vi "AnalogCNTL_MKS.vi"() -> ()   [LabVIEW 2015]
uses:
  <userlib>/caLab/Private/Get_PV-1D.vi
panel:
  in  "LocalEpics":u16(ring) items=["LOCAL", "EPCIS"]
  out "APX:HPC100":dbl format="%.3g"
  out "APX:HPC01":dbl format="%_6g"
  out "Gain":dbl format="%#_6f"
  out "Vin":dbl
  in  "Vref":dbl min=0.0 max=5.0 step=0.01
  in  "ManualAuto":u16(ring) items=["CLOSE", "OPEN", "AUTO"]
  in  "MFC0:Pcell_RQ":dbl
  out "MFC0:Pcell":dbl
  in  "stop":bool
  # "MFC0"
  # "MFC"
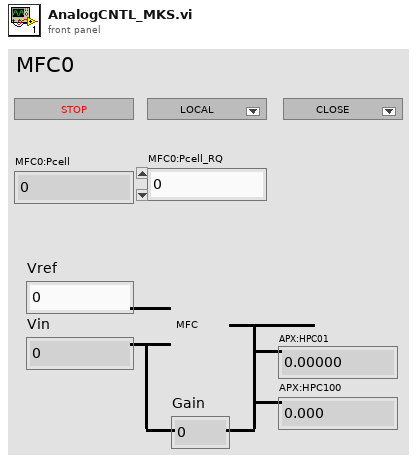
[diagram p1: front panel]
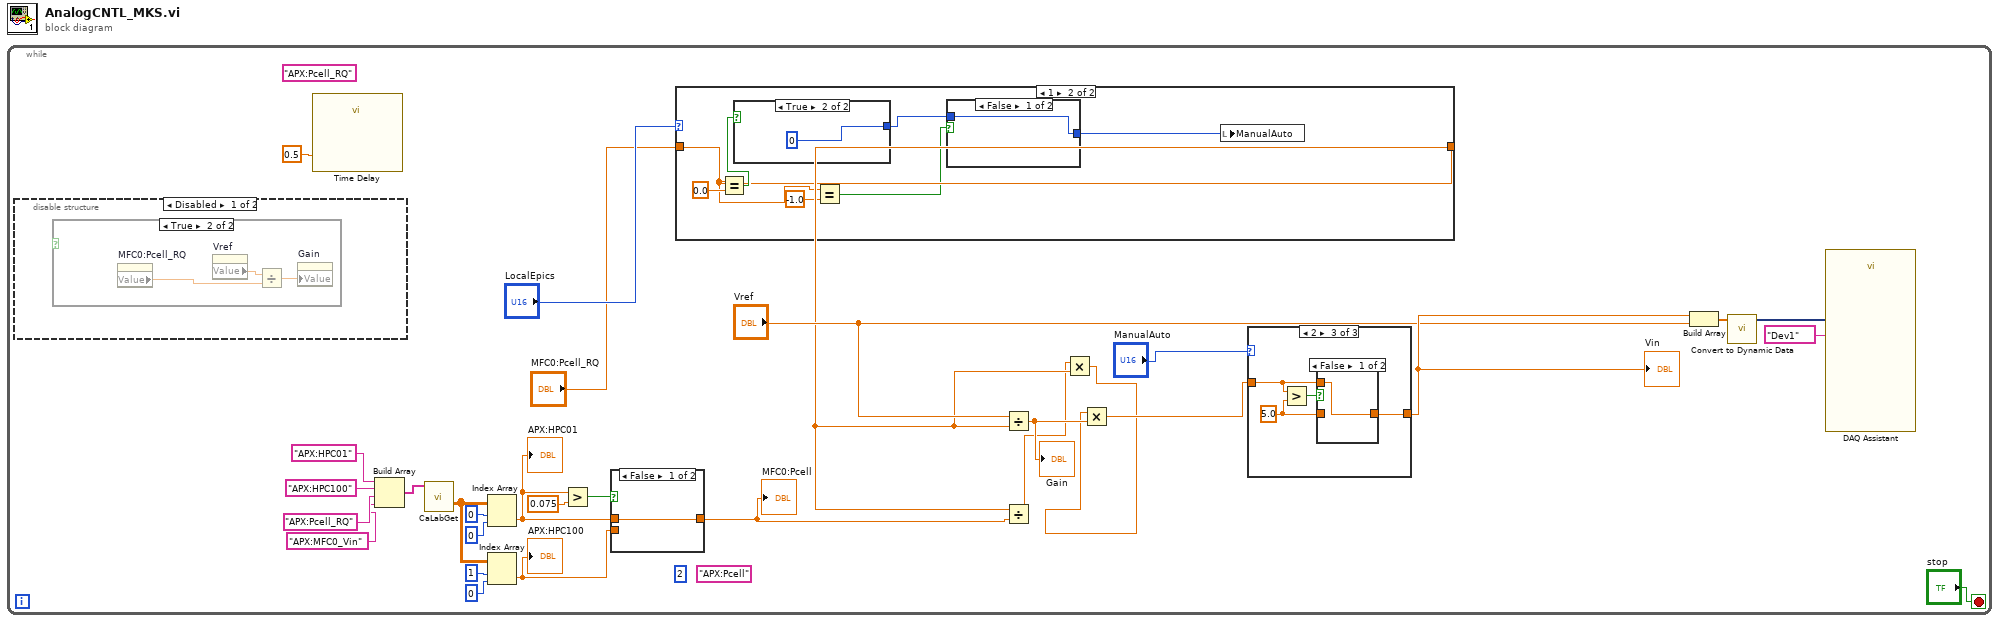
[diagram p0: block diagram]
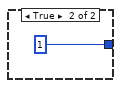
[diagram p4: hidden frame]
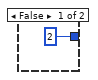
[diagram p5: hidden frame]
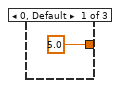
[diagram p8: hidden frame]
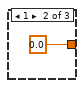
[diagram p9: hidden frame]
diagram:
  n1 = while {
    stop <- "stop" stop-if-true
    (unwired) "APX:Pcell"
    (unwired) "APX:Pcell_RQ"
    (unwired) u16 2 ("y")
    n2 = disable-structure shown="Disabled" {
      frame Disabled {
        n3 = case shown="True" {
          selector: _ -> [_ _]
          frame False {
          }
          frame True {
            n4 = property on="MFC0:Pcell_RQ" class="DigNum (strict)"() -> ("Value"=w45:dbl)  [unwired: 2 in, 2 out]
            n5 = property on="Vref" class="DigNum (strict)"() -> ("Value"=w46:dbl)  [unwired: 2 in, 2 out]
            n6 = Divide(x=w46, y=w45) -> (x/y=w47:dbl)
            n7 = property on="Gain" class="DigNum (strict)"("Value"=w47) -> ()  [unwired: 2 in, 2 out]
          }
        }
      }
      frame Enabled {
      }
    }
    n8 = call "Time Delay"("Delay Time (s)"=0.5) -> ()  [unwired: 10 in, 1 out]
    n9 = Build Array("APX:HPC01", "APX:HPC100", "APX:Pcell_RQ", "APX:MFC0_Vin") -> (w24:string[])
    n10 = call-poly "CaLabGet.vi"("PV Names"=w24) -> ("Value Array (number)"=w20:dbl[][])  [unwired: 8 in, 6 out]
    n11 = Index Array(array=w20, index (row)=0 ("disabled index (col)"), index (col)=0) -> (element=w10:dbl)
    "APX:HPC01" <- w10
    n12 = Index Array(array=w20, index (row)=1 ("disabled index (col)"), index (col)=0) -> (element=w11:dbl)
    "APX:HPC100" <- w11
    n13 = Greater?(x=w10, y=0.075) -> (0:w13:bool)
    n14 = case shown="False" w13 {
      tunnel: w11 -> [_ w32]
      tunnel: [w31 w32] -> w5
      tunnel: w10 -> [w31 _]
      frame False {
      }
      frame True {
      }
    }
    "MFC0:Pcell" <- w5
    n15 = case shown="1" "LocalEpics" {
      tunnel: "MFC0:Pcell_RQ" -> [w33 w37]
      tunnel: [w33 w37] -> w3
      frame 0, Default {
      }
      frame 1 {
        n16 = Equal?(x=w37, y=0.0) -> (x = y?=w38:bool)
        n17 = case shown="True" w38 {
          tunnel: [u16 2 ("ManualAuto") u16 0 ("ManualAuto")] -> w35
          frame False {
          }
          frame True {
          }
        }
        n18 = Equal?(x=w37, y=-1.0) -> (x = y?=w36:bool)
        n19 = case shown="False" w36 {
          tunnel: w35 -> [w41 _]
          tunnel: [w41 1] -> w34
          frame False {
          }
          frame True {
          }
        }
        n20 = local write "ManualAuto"(w34) -> ()
      }
    }
    n21 = Divide(x="Vref", y=w3) -> (x/y=w15:dbl)
    "Gain" <- w15
    n22 = Divide(x=w3, y=w5) -> (x/y=w2:dbl)
    n23 = Multiply(x=w2, y=w3) -> (x*y=w1:dbl)
    n24 = Multiply(x=w1, y=w15) -> (x*y=w27:dbl)
    n25 = case shown="2" "ManualAuto" {
      tunnel: [5.0 ("APX:MFC0_Vin") 0.0 ("APX:MFC0_Vin") w51] -> w16
      tunnel: w27 -> [_ _ w52]
      frame 0, Default {
      }
      frame 1 {
      }
      frame 2 {
        w50 = 5.0 ("y")
        n26 = Greater?(x=w52, y=w50) -> (0:w53:bool)
        n27 = case shown="False" w53 {
          tunnel: w52 -> [w54 _]
          tunnel: [w54 w55] -> w51
          tunnel: w50 -> [_ w55]
          frame False {
          }
          frame True {
          }
        }
      }
    }
    "Vin" <- w16
    n28 = Build Array(w16, "Vref") -> (w17:dbl[])
    n29 = call "Convert to Dynamic Data"("Array"=w17) -> ("Dynamic Data Type"=w28:dynamicdata)  [unwired: 3 in]
    n30 = call "DAQ Assistant"("data"=w28, "device name"=tag "Dev1") -> ()  [unwired: 16 in, 2 out]
  }
